vi "zadanie3.vi"() -> ()   [LabVIEW 2012]
panel:
  out "Wartoœæ temperatury w st C:":dbl
  out "Wartoœæ temperatury w st K":dbl
  in  "Rozpocznij":bool
  in  "Podaj potencja³ elektrokinetyczny (mV):":dbl
  # "Program oblicza temperaturê na podstawie podanego potencja³u elektrokinetycznego:"
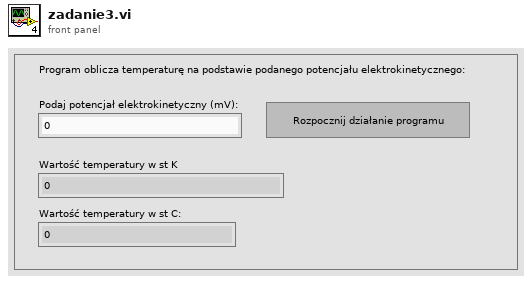
[diagram p1: front panel]
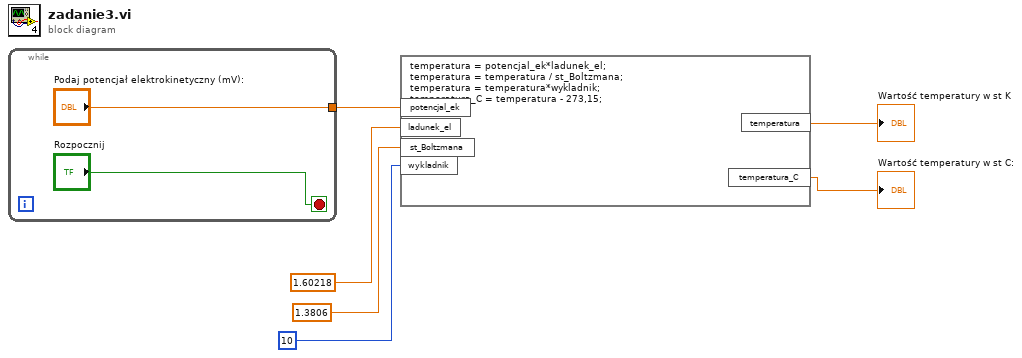
[diagram p0: block diagram]
diagram:
  n1 = while {
    tunnel: ["Podaj potencja³ elektrokinetyczny (mV):"] -> w5
    stop <- "Rozpocznij" stop-if-true
  }
  n2 = formula code="temperatura = potencjal_ek*ladunek_el;\ntemperatura = temperatura / st_Boltzmana;\ntemperatura = temperatura*wykladnik;\ntemperatura_C = temperatura - 273,15;"("potencjal_ek"=w5, "ladunek_el"=1.60218, "st_Boltzmana"=1.3806, "wykladnik"=10) -> ("temperatura"=→"Wartoœæ temperatury w st K":dbl, "temperatura_C"=→"Wartoœæ temperatury w st C:":dbl)
